vi "Calculate 3dB RC.vi"(10 "filter order":i32, 11 "time constant (s)":dbl) -> (3 "f -3 dB (Hz)":dbl)   [LabVIEW 2019, in "DSP.lvclass"]
uses:
  DSP.lvclass
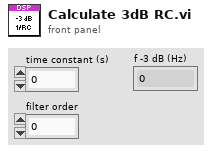
[diagram p1: front panel]
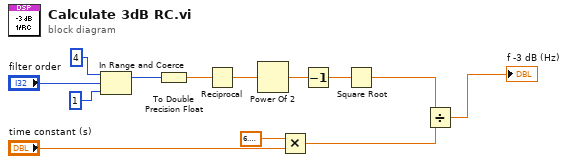
[diagram p0: block diagram]
diagram:
  n1 = In Range and Coerce(upper limit=4 ("lower limit"), x="filter order", lower limit=1) -> (coerced(x)=w3:i32)  [unwired: 1 out]
  n2 = To Double Precision Float(number=w3) -> (double precision float=w10:dbl)
  n3 = Reciprocal(x=w10) -> (1/x=w9:dbl)
  n4 = Power Of 2(x=w9) -> (2^x=w11:dbl)
  n5 = Multiply(x=6.283185307179586, y="time constant (s)") -> (x*y=w7:dbl)
  n6 = Decrement(x=w11) -> (x-1=w8:dbl)
  n7 = Square Root(x=w8) -> (sqrt(x)=w2:dbl)
  n8 = Divide(x=w2, y=w7) -> (x/y=→"f -3 dB (Hz)":dbl)
